vi "TRITON_TEMP_CONTROL_STABILITY_EXAMPLE.vi"() -> ()   [LabVIEW 2009]
panel:
  out "RI Response":string
  in  "Heater Control Mode":enum16{"Open Loop", "Closed Loop"}(ring)=enum."Closed Loop"
  in  "Heater Range":dbl
  out "Connection Open":bool
  in  "Target Temperature [K]":dbl
  in  "D":dbl
  in  "I":dbl=300.0
  in  "P":dbl=10.0
  in  "Temperature Control Channel":i32=5
  out "Locked?":bool
  out "Current Temperature [K]":dbl
  in  "Array length to monitor":i32=60
  out "Temperature Vs Time Plot":cluster{dbl[], dbl[]}(graph)
  out "Elapsed Time in Seconds":dbl
  in  "stop":bool
  in  "Start Monitoring":bool
  out "error out":errorcluster
  in  "error in (no error)":errorcluster
  in  "Open Connection":bool
  in  "Timeout":i32=10000
  in  "Remote Port":i32=33576
  in  "IP Address":string
  in  "Bytes to Read":i32=5000
  in  "Mode":T1(ring)=enum."Immediate"
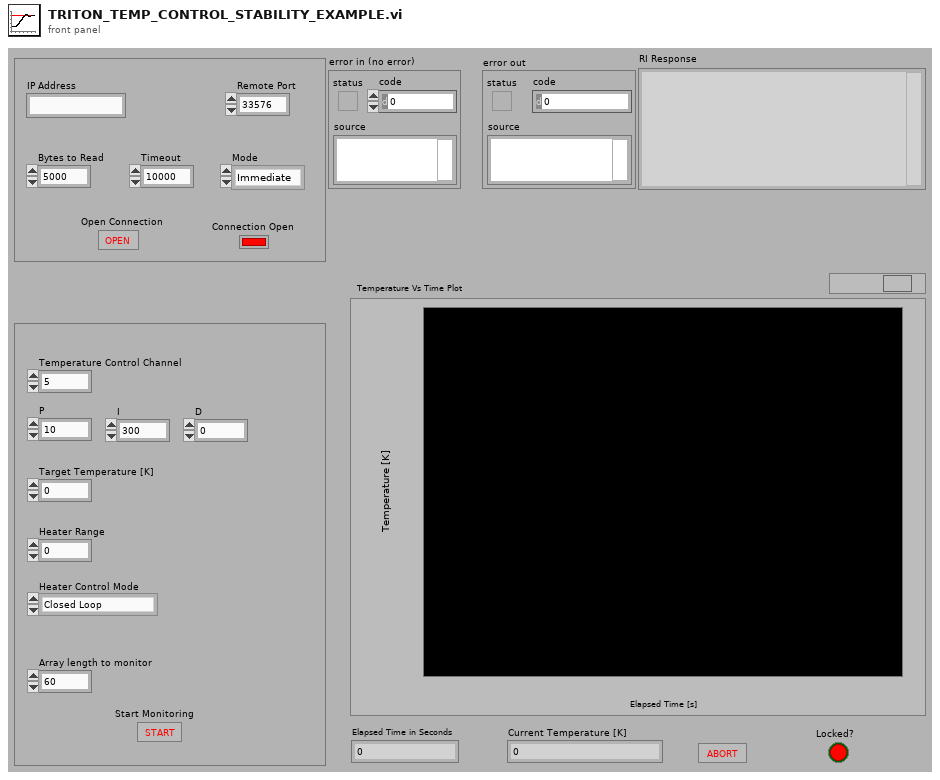
[diagram p1: front panel]
types:
  T1 = enum16{"Standard", "Buffered", "CRLF", "Immediate"}
  T2 = cluster{"Mode":enum16{"Standard", "Buffered", "CRLF", "Immediate"}, "Bytes to Read":i32, "IP Address":string, "Remote Port":i32, "Timeout":i32}
  T3 = cluster{"Mode":enum16{"Standard", "Buffered", "CRLF", "Immediate"}, "Bytes to Read":i32, "IP Address":string, "Remote Port":i32, "Timeout":i32, "connection ID":refnum<k5>}
  T4 = cluster{"Updated array":dbl[], "Updated array":dbl[]}
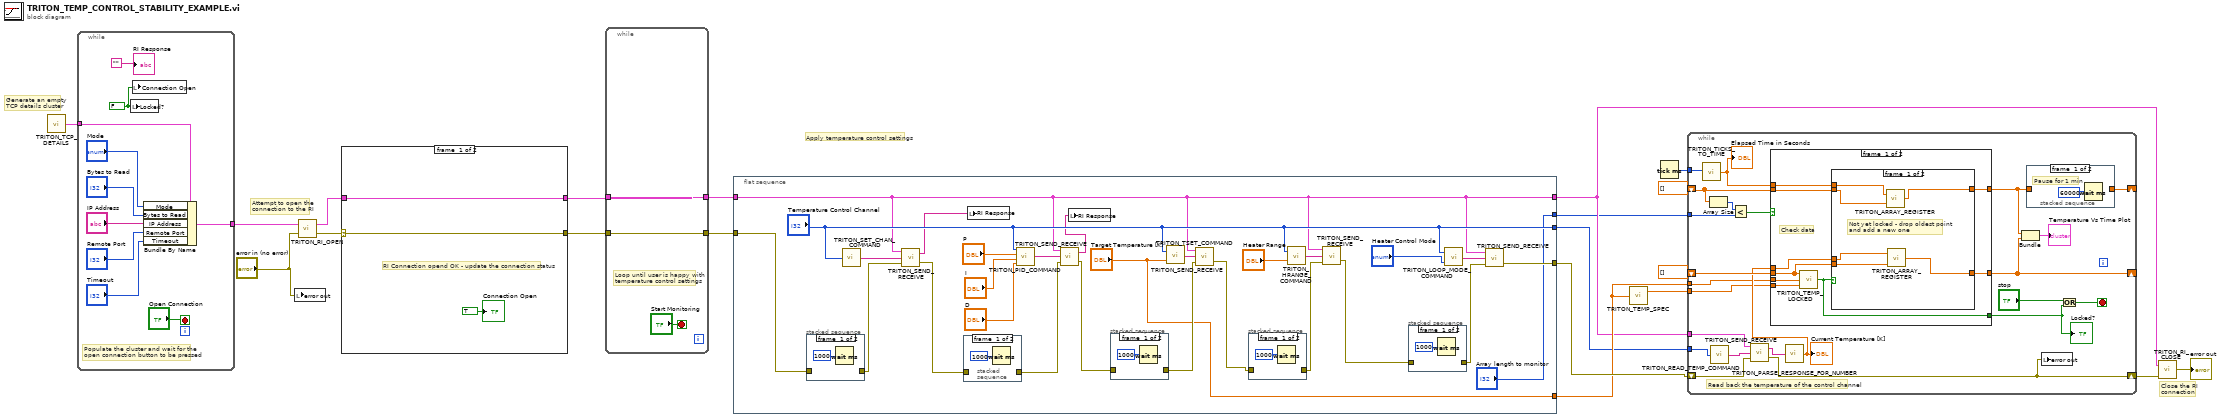
[diagram p0: block diagram]
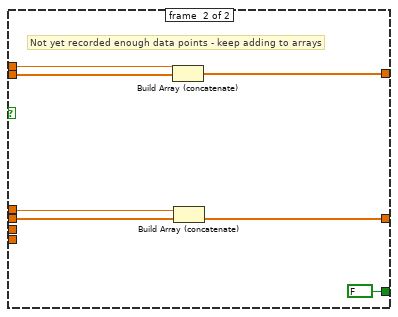
[diagram p8: hidden frame]
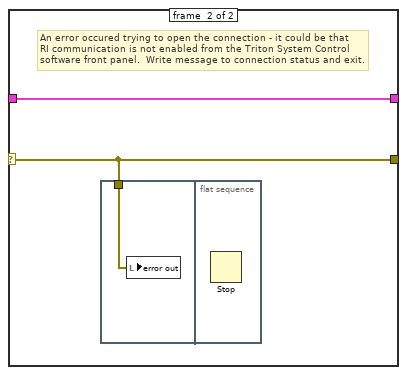
[diagram p10: hidden frame]
diagram:
  # "Apply temperature control settings"
  # "Close the RI\nconnection"
  # "Attempt to open the\nconnection to the RI"
  # "Generate an empty\nTCP details cluster"
  n1 = call "TRITON_TCP_DETAILS.vi"() -> ("Cluster"=w20:T2)
  n2 = while {
    tunnel: w20 -> [w30]
    tunnel: [w23] -> w15
    stop <- "Open Connection" stop-if-true
    w22 = FALSE ("Locked?")
    # "Populate the cluster and wait for the\nopen connection button to be pressed"
    n3 = local write "Locked?"(w22) -> ()
    n4 = local write "Connection Open"(w22) -> ()
    n5 = Bundle By Name(cluster=w30, "Mode"="Mode", "Bytes to Read"="Bytes to Read", "IP Address"="IP Address", "Remote Port"="Remote Port", "Timeout"="Timeout") -> (w23:T2)
    "RI Response" <- ""
  }
  n6 = local write "error out"("error in (no error)") -> ()
  n7 = call "TRITON_RI_OPEN.vi"("error in (no error)"="error in (no error)", "Cluster"=w15) -> ("error out"=w17:errorcluster, "output cluster"=w19:T3)
  n8 = case shown="No Error" w17 {
    selector: w17 -> [w32 w34]
    tunnel: w19 -> [w33 w35]
    tunnel: [w33 w35] -> w14
    tunnel: [w32 w34] -> w13
    frame #0 {
      # "RI Connection opend OK - update the connection status"
      "Connection Open" <- TRUE ("Connection Open")
    }
    frame #1 {
      # "An error occured trying to open the connection - it could be that\nRI communication is not enabled from the Triton System Control\nsoftware front panel.  Write message to connection status and exit."
      n9 = flat-sequence {
        tunnel: w34 -> [w36]
        frame #0 {
          n10 = local write "error out"(w36) -> ()
        }
        frame #1 {
          n11 = Stop() -> ()  [unwired: 1 in]
        }
      }
    }
  }
  n12 = while {
    tunnel: w14 -> [w37]
    tunnel: w13 -> [w38]
    tunnel: [w38] -> w7
    tunnel: [w37] -> w4
    stop <- "Start Monitoring" stop-if-true
    # "Loop until user is happy with\ntemperature control settings"
  }
  n13 = flat-sequence {
    tunnel: w7 -> [w60]
    tunnel: [w46] -> w6
    tunnel: ["Target Temperature [K]"] -> w5
    tunnel: w4 -> [w43]
    tunnel: ["Temperature Control Channel"] -> w3
    tunnel: [w43] -> w2
    tunnel: ["Array length to monitor"] -> w1
    frame #0 {
      n14 = stacked-sequence {
        tunnel: w60 -> [_ w76]
        tunnel: [_ w76] -> w59
        frame #0 {
          n15 = Wait (ms)(milliseconds to wait=u32 1000) -> ()  [unwired: 1 out]
        }
        frame #1 {
        }
      }
      n16 = call "TRITON_SET_CHAN_COMMAND.vi"("Temperature Control Channel"="Temperature Control Channel") -> ("Command String"=w66:string)
      n17 = call "TRITON_SEND_RECEIVE.vi"("error in (no error)"=w59, "Command String"=w66, "Communication Cluster"=w43) -> ("error out"=w58:errorcluster, "Response String"=w40:string)
      n18 = stacked-sequence {
        tunnel: w58 -> [_ w74]
        tunnel: [_ w74] -> w57
        frame #0 {
          n19 = Wait (ms)(milliseconds to wait=u32 1000) -> ()  [unwired: 1 out]
        }
        frame #1 {
        }
      }
      n20 = local write "RI Response"(w40) -> ()
      n21 = call "TRITON_PID_COMMAND.vi"("D"="D", "I"="I", "P"="P", "Control Channel"="Temperature Control Channel") -> ("PID Command"=w62:string)
      n22 = call "TRITON_SEND_RECEIVE.vi"("error in (no error)"=w57, "Command String"=w62, "Communication Cluster"=w43) -> ("error out"=w56:errorcluster, "Response String"=w41:string)
      n23 = local write "RI Response"(w41) -> ()
      n24 = stacked-sequence {
        tunnel: w56 -> [_ w72]
        tunnel: [_ w72] -> w55
        frame #0 {
          n25 = Wait (ms)(milliseconds to wait=u32 1000) -> ()  [unwired: 1 out]
        }
        frame #1 {
        }
      }
      n26 = call "TRITON_TSET_COMMAND.vi"("Target Temperature [K]"="Target Temperature [K]", "Temperature Control Channel"="Temperature Control Channel") -> ("Command String"=w61:string)
      n27 = call "TRITON_SEND_RECEIVE.vi"("error in (no error)"=w55, "Command String"=w61, "Communication Cluster"=w43) -> ("error out"=w52:errorcluster)  [unwired: 1 out]
      n28 = stacked-sequence {
        tunnel: w52 -> [_ w70]
        tunnel: [_ w70] -> w51
        frame #0 {
          n29 = Wait (ms)(milliseconds to wait=u32 1000) -> ()  [unwired: 1 out]
        }
        frame #1 {
        }
      }
      n30 = call "TRITON_HRANGE_COMMAND.vi"("Heater Range [A]"="Heater Range", "Temperature Control Channel"="Temperature Control Channel") -> ("Command String"=w53:string)
      n31 = call "TRITON_SEND_RECEIVE.vi"("error in (no error)"=w51, "Command String"=w53, "Communication Cluster"=w43) -> ("error out"=w48:errorcluster)  [unwired: 1 out]
      n32 = stacked-sequence {
        tunnel: w48 -> [_ w68]
        tunnel: [_ w68] -> w47
        frame #0 {
          n33 = Wait (ms)(milliseconds to wait=u32 1000) -> ()  [unwired: 1 out]
        }
        frame #1 {
        }
      }
      n34 = call "TRITON_LOOP_MODE_COMMAND.vi"("Heater Control Mode"="Heater Control Mode", "Temperature Control Channel"="Temperature Control Channel") -> ("Command String"=w49:string)
      n35 = call "TRITON_SEND_RECEIVE.vi"("error in (no error)"=w47, "Command String"=w49, "Communication Cluster"=w43) -> ("error out"=w46:errorcluster)  [unwired: 1 out]
    }
  }
  n36 = call "TRITON_TEMP_SPEC.vi"("Target Temperature [K]"=w5) -> ("Temperature Stability Specification"=w9:dbl)
  n37 = Tick Count (ms)() -> (millisecond timer value=w12:u32)
  n38 = while {
    tunnel: w12 -> [w99]
    shift-right: [w97] -> _
    shift-left: dbl[] [] -> [w87]
    shift-right: [w95] -> _
    shift-left: dbl[] [] -> [w96]
    shift-right: [w91] -> w8
    shift-left: w6 -> [w92]
    tunnel: w1 -> [w85]
    tunnel: w9 -> [w82]
    tunnel: w3 -> [w78]
    tunnel: w2 -> [w79]
    tunnel: w5 -> [w77]
    stop <- w90 stop-if-true
    # "Read back the temperature of the control channel"
    n39 = call "TRITON_TICKS_TO_TIME.vi"("Initial millisecond timer value"=w99) -> ("Elapsed Time in Seconds"=w98:dbl)
    "Elapsed Time in Seconds" <- w98
    n40 = Array Size(array=w87) -> (size(s)=w86:i32)
    n41 = call "TRITON_READ_TEMP_COMMAND.vi"("Temperature Channel"=w78) -> ("Command String"=w89:string)
    n42 = Less?(x=w86, y=w85) -> (x < y?=w84:bool)
    n43 = call "TRITON_SEND_RECEIVE.vi"("error in (no error)"=w92, "Command String"=w89, "Communication Cluster"=w79) -> ("error out"=w91:errorcluster, "Response String"=w88:string)
    n44 = call "TRITON_PARSE_RESPONSE_FOR_NUMBER.vi"("Input String"=w88) -> ("Output"=w83:dbl)
    "Current Temperature [K]" <- w83
    n45 = case shown="False" w84 {
      tunnel: w98 -> [w102 w123]
      tunnel: w96 -> [w104 w122]
      tunnel: [w105 w121] -> w95
      tunnel: [w107 w120] -> w94
      tunnel: w87 -> [w106 w119]
      tunnel: w83 -> [w103 w118]
      tunnel: w82 -> [w108 _]
      tunnel: [w101 FALSE ("Locked on Setpoint?")] -> w80
      tunnel: w77 -> [w100 _]
      frame #0 {
        # "Check data"
        n46 = call "TRITON_TEMP_LOCKED.vi"("Temperature Control Spec"=w108, "Target Temperature"=w100, "Temperature Data Array"=w104) -> ("Locked on Setpoint?"=w101:bool)
        n47 = case shown="False" w101 {
          tunnel: [w110 w116] -> w107
          tunnel: w106 -> [w111 w116]
          tunnel: [w112 w115] -> w105
          tunnel: w104 -> [w114 w115]
          tunnel: w103 -> [w113 _]
          tunnel: w102 -> [w109 _]
          frame #0 {
            # "Not yet locked - drop oldest point\nand add a new one"
            n48 = call "TRITON_ARRAY_REGISTER.vi"("Input array"=w111, "New value"=w109) -> ("Updated array"=w110:dbl[])
            n49 = call "TRITON_ARRAY_REGISTER.vi"("Input array"=w114, "New value"=w113) -> ("Updated array"=w112:dbl[])
          }
          frame #1 {
            # "Temperature locked - stop adding\ndata and exit loop"
          }
        }
      }
      frame #1 {
        # "Not yet recorded enough data points - keep adding to arrays"
        n50 = Build Array (concatenate)(w123, w119) -> (w120:dbl[])
        n51 = Build Array (concatenate)(w118, w122) -> (w121:dbl[])
      }
    }
    "Locked?" <- w80
    n52 = Bundle("Updated array"=w94, "Updated array"=w95) -> (→"Temperature Vs Time Plot":T4)  [unwired: 1 in]
    n53 = stacked-sequence {
      tunnel: w94 -> [_ w125]
      tunnel: [_ w125] -> w97
      frame #0 {
        # "Pause for 1 min"
        n54 = Wait (ms)(milliseconds to wait=u32 60000) -> ()  [unwired: 1 out]
      }
      frame #1 {
      }
    }
    n55 = local write "error out"(w91) -> ()
    n56 = Or(x="stop", y=w80) -> (x .or. y?=w90:bool)
  }
  n57 = call "TRITON_RI_CLOSE.vi"("error in (no error)"=w8, "Communication Cluster"=w2) -> ("error out"=→"error out":errorcluster)
